vi "IRISS_FPGA_IO_v4.vi"() -> ()   [LabVIEW 2016]
doc: "This VI contains a basic quadrature decoder which is reset asynchronously upon clicking the reset button."
uses:
  <vilib>/Platform/TimedLoop/XDataNode/timing_clust.ctl
  <vilib>/Platform/TimedLoop/XDataNode/nitl_modes.ctl
  <vilib>/Platform/TimedLoop/XDataNode/wakeup.ctl
  <vilib>/rvi/Emulation/niFpgaGetClockAttributes.vi
  <vilib>/rvi/Emulation/niFpgaSctlEmulationGetInTimedLoop.vi
  <vilib>/rvi/Emulation/niFpgaEmulationReportErrorSimple.vi
  <vilib>/rvi/eio/common/nirviEmuTemplateMethod_errors.vi
  <vilib>/rvi/Emulation/niFpgaCriticalErrorInLSC.vi
  <vilib>/eio/EIONode/EIONode.xnode
  <vilib>/platform/TimedLoop/XDataNode/XDataNode.xnode
  <vilib>/Platform/TimedLoop/XDataNode/XDNodeRunTimeDep.lvlib
  Library/KevinLibraryAll/labview/KevLib01.lvlib
  Library/jmslib.lvlib
panel:
  in  "Connector2/DIO7":bool
  in  "Connector2/DIO8":bool
  in  "Connector2/DIO9":bool
  in  "Connector2/DIO10":bool
  in  "PWM1":fxp<+,32,0>
  in  "Period 1 (Ticks)":u32=1000
  in  "Period (Ticks)":u32=2000
  in  "DIR OCT Mot":bool
  in  "INHB OCT Mot":bool
  out "FAULT OCT Mot":bool
  out "Position OCT Mot":i32
  out "JumpBy2Error OCT Mot":i16
  in  "Reset OCT Mot":bool
  in  "OCT Mot DC":fxp<+,32,0>
  in  "Conn0/DIO15 Button 4":bool
  in  "Conn0/DIO12 Button 1":bool
  in  "Conn0/DIO13 Button 2":bool
  out "Home OCT z":bool
  in  "DIR Y":bool
  in  "INHB Y":bool
  out "FAULT Y":bool
  out "Position Y":i32
  out "JumpBy2Error Y":i16
  in  "Reset Y":bool
  in  "Y DC":fxp<+,32,0>
  in  "DIR X":bool
  in  "INHB X":bool
  out "FAULT X":bool
  out "Position X":i32
  out "JumpBy2Error X":i16
  in  "Reset X":bool
  in  "DIR Z":bool
  in  "INHB Z":bool
  out "FAULT Z":bool
  out "Position Z":i32
  out "JumpBy2Error Z":i16
  in  "Reset Z":bool
  in  "Z DC":fxp<+,32,0>
  in  "X DC":fxp<+,32,0>
  out "samples":i32
  out "Current Monitor":u32[](array[numeric])
  out "Raw Data Response (MSB)":bool[](array[boolean])
  out "Home L4":bool
  out "Home L1":bool
  out "Home L2":bool
  out "Home L3":bool
  in  "Positive Direction C1-4":bool
  out "JumpBy2Error C1-4":i16
  out "32 bit Position C1-4":i32
  in  "Reset C1-4":bool
  in  "Positive Direction C1-1":bool
  out "JumpBy2Error C1-1":i16
  out "32 bit Position C1-1":i32
  in  "Reset C1-1":bool
  out "32 bit Position 17":i32
  in  "Reset 17":bool
  in  "Positive Direction 17":bool
  out "JumpBy2Error 17":i16
  out "32 bit Position 16":i32
  in  "Reset 16":bool
  in  "Positive Direction 16":bool
  out "JumpBy2Error 16":i16
  out "32 bit Position 15":i32
  in  "Reset 15":bool
  in  "Positive Direction 15":bool
  out "JumpBy2Error 15":i16
  out "32 bit Position 14":i32
  in  "Reset 14":bool
  in  "Positive Direction 14":bool
  out "JumpBy2Error 14":i16
  out "32 bit Position 13":i32
  in  "Reset 13":bool
  in  "Positive Direction 13":bool
  out "JumpBy2Error 13":i16
  out "32 bit Position 12":i32
  in  "Reset 12":bool
  in  "Positive Direction 12":bool
  out "JumpBy2Error 12":i16
  out "32 bit Position 11":i32
  in  "Reset 11":bool
  in  "Positive Direction 11":bool
  out "JumpBy2Error 11":i16
  out "32 bit Position 10":i32
  in  "Reset 10":bool
  in  "Positive Direction 10":bool
  out "JumpBy2Error 10":i16
  out "32 bit Position 9":i32
  in  "Reset 9":bool
  in  "Positive Direction 9":bool
  out "JumpBy2Error 9":i16
  out "JumpBy2Error 3":i16
  in  "Positive Direction 3":bool
  out "JumpBy2Error 1":i16
  in  "Positive Direction 1":bool
  out "AI":i16[](array[numeric])
  out "32 bit Position 3":i32
  in  "Reset 3":bool
  in  "AO":i16[](array[numeric])=[0, 0, 0, 0, 0, 0, 0, 0]
  out "32 bit Position 1":i32
  in  "Reset 1":bool
  # "Accurus Buttons"
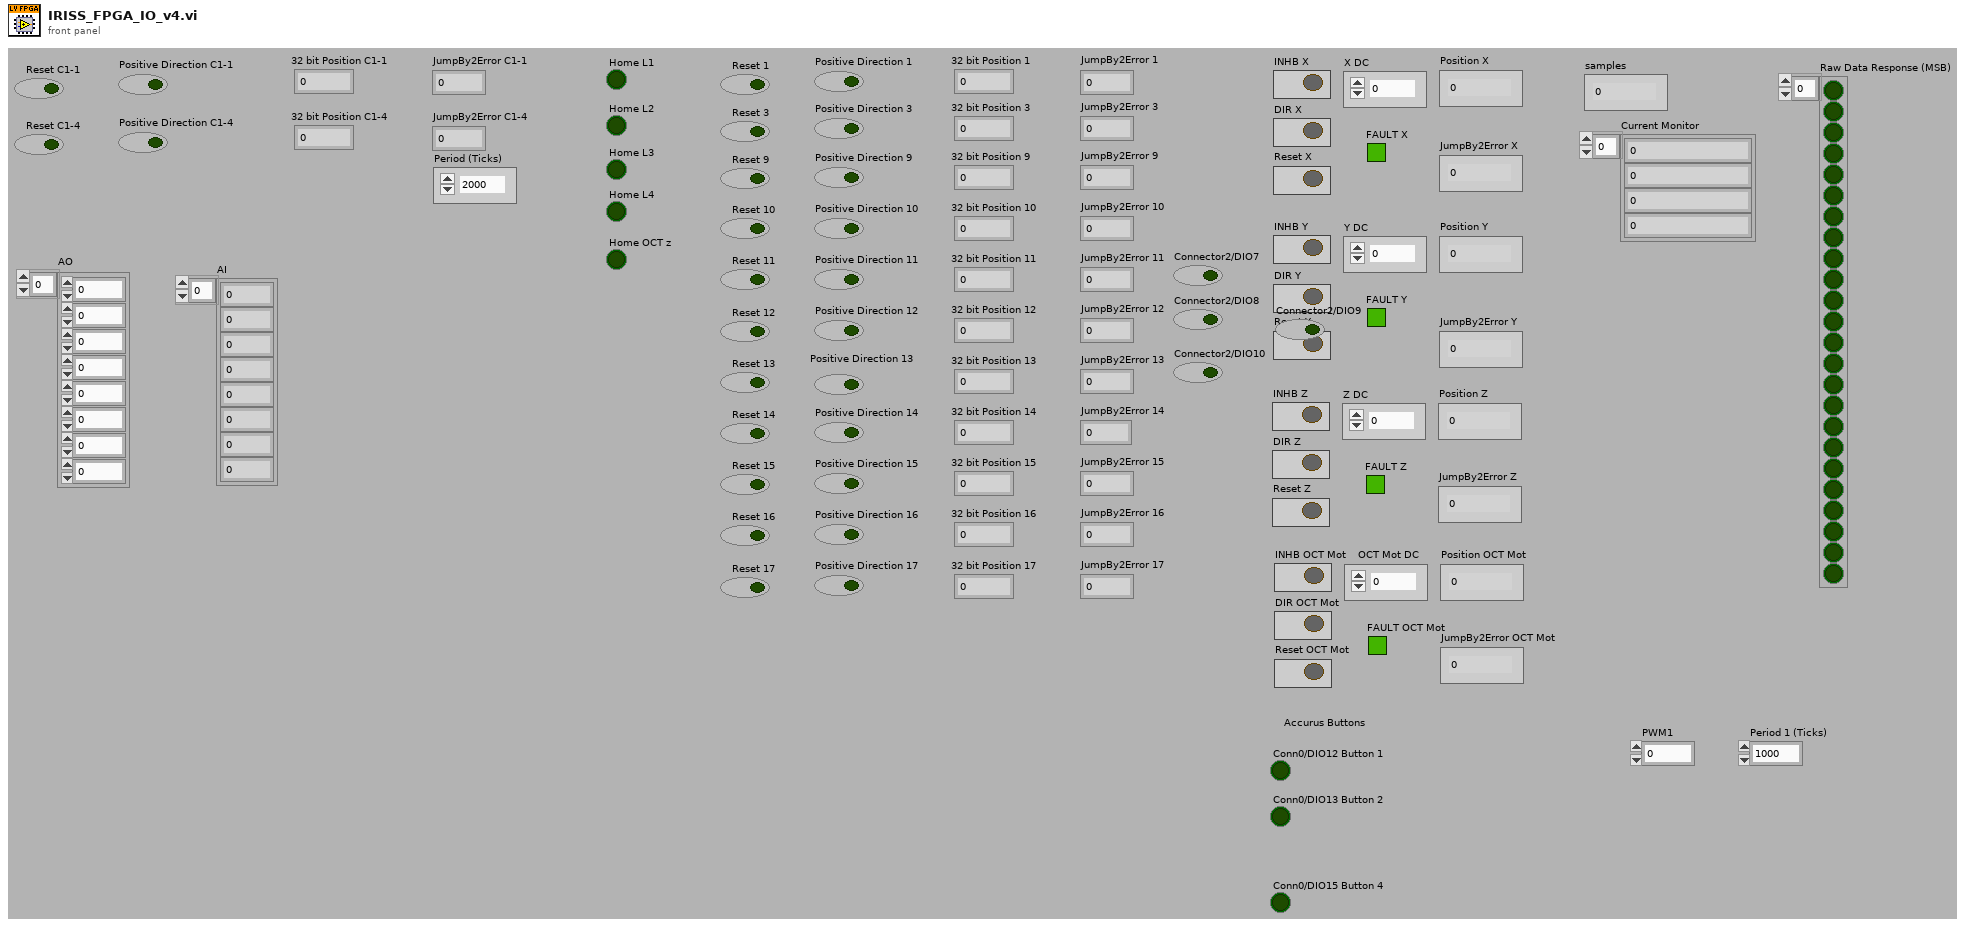
[diagram p1: front panel]
types:
  T1 = typedef "XDNodeRunTimeDep.lvlib/timing_clust.ctl" = cluster{"Expected End [f-1]":u64, "Actual End [f-1]":u64, "Finished Late? [f-1]":bool, "Expected End [i-1]":u64, "Actual End [i-1]":u64, "Finished Late? [i-1]":bool, "Expected Start [i]":u64, "Actual Start [i]":u64, "Expected Start [f]":u64, "Actual Start [f]":u64, "Source Name":string, "Structure Name":string, "Period":i64, "Deadline":i64, "Offset":i64, "Start":i64, "Priority":i32, "Timeout":i32, "Mode":T2, "Wakeup Reason":T3, "Error":errorcluster, "Source Type":string, "Secondary Source Type":string, "Global End Time":u64, "Global Start Time":u64, "Frame Duration":u64, "Iteration Duration":u64, "Assigned CPU":i32, "I/O Scan Engine Mode":u32}
  T2 = typedef "XDNodeRunTimeDep.lvlib/nitl_modes.ctl" = enum32{"No Change", "Process missed periods, maintain original phase", "Discard missed periods, maintain original phase", "Process missed periods, ignore original phase", "Discard missed periods, ignore original phase"}
  T3 = typedef "XDNodeRunTimeDep.lvlib/wakeup.ctl" = enum32{"Normal", "Aborted", "Asynchronous wakeup", "Timing source error", "Timed loop error", "Timeout"}
  T4 = cluster{"PWM In":refnum<k21>, "Direction":refnum<k21>, "Inhibit":refnum<k21>, "Encoder C":refnum<k21>, "Encoder B":refnum<k21>, "Encoder A":refnum<k21>, "Fault":refnum<k21>}
  T5 = cluster{"SCLK":refnum<k21>, "MOSI":refnum<k21>, "MISO":refnum<k21>}
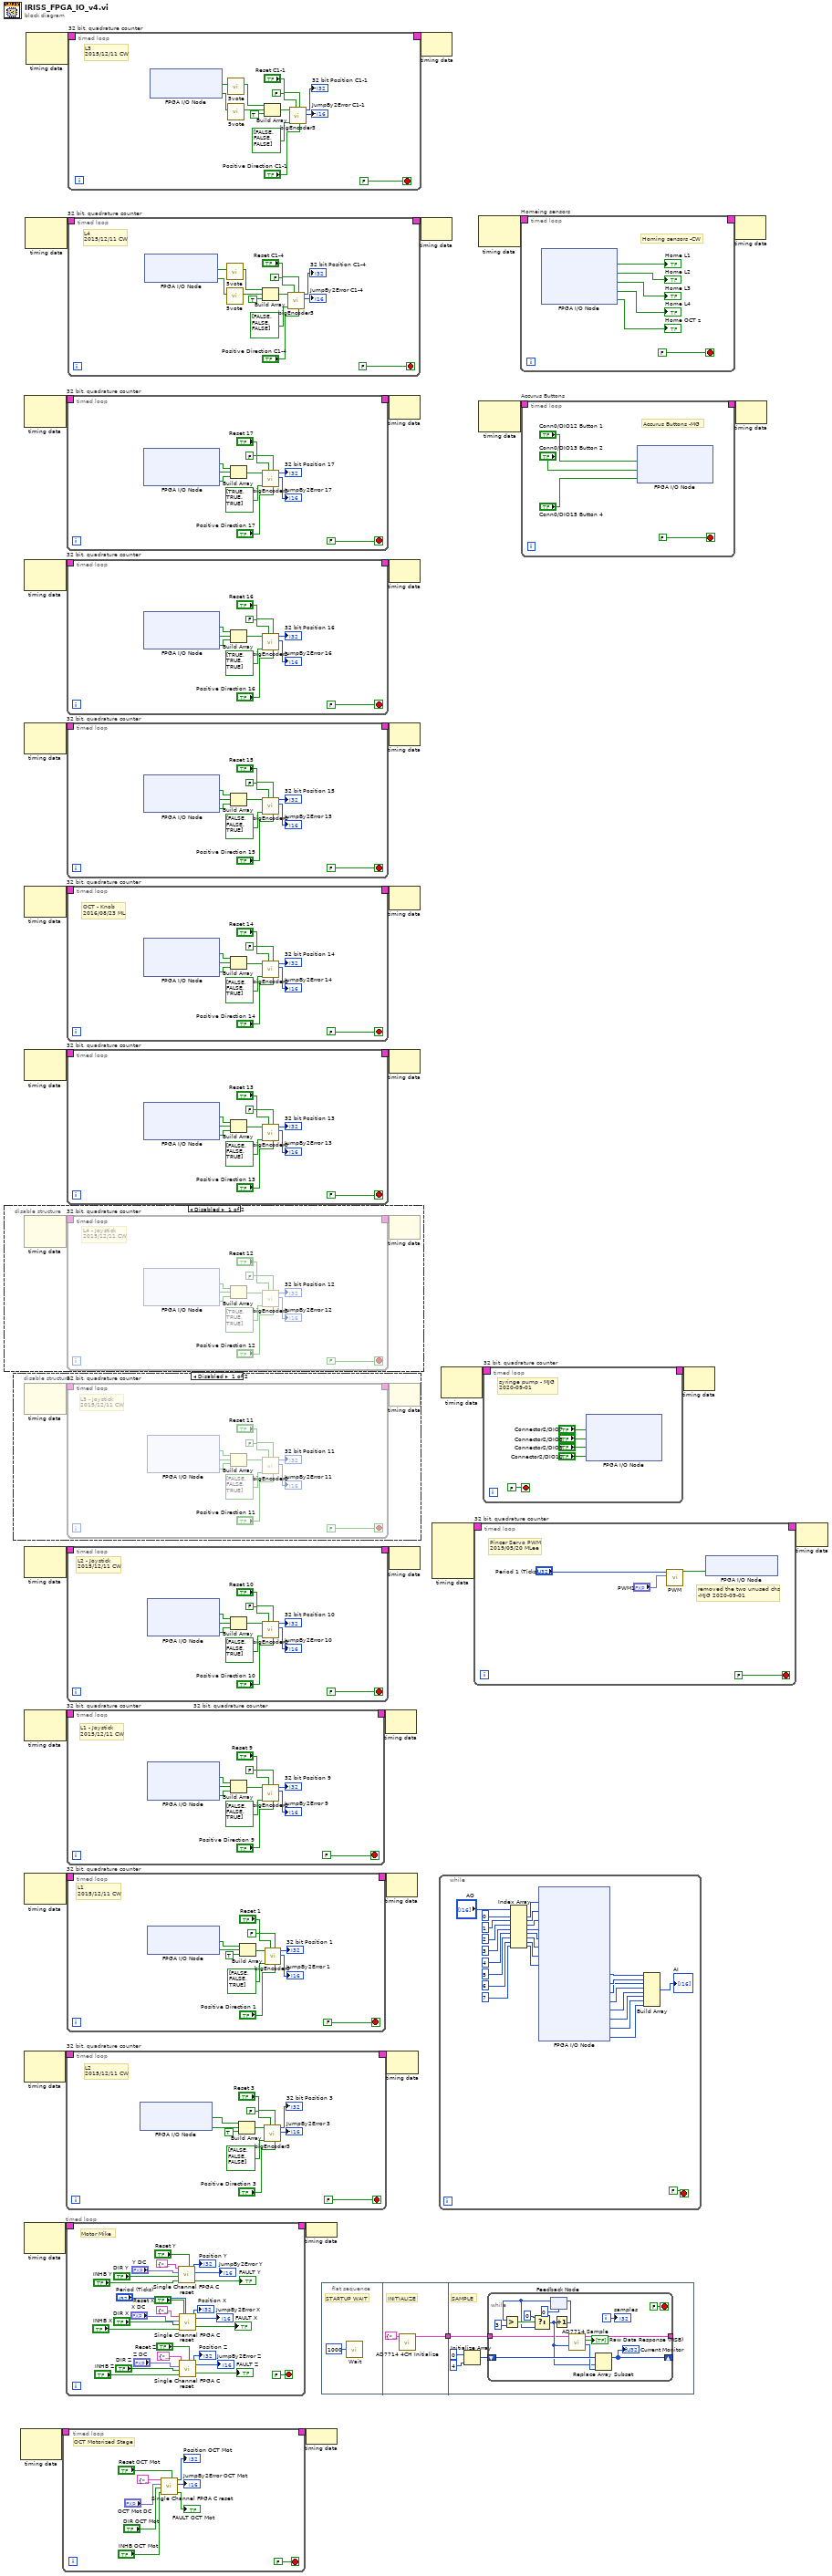
[diagram p0: block diagram]
diagram:
  n1 = disable-structure shown="Disabled" {
    frame Disabled {
      n2 = node-c288() -> (w37:T1)  [unwired: 2 out]
      n3 = timed-loop "32 bit, quadrature counter" {
        timing-out: [_] -> w36
        timing: w37 -> [_]
        stop <- FALSE stop-if-true
        # "L4 - Joystick\n2015/12/11 CW"
        n4 = xnode "FPGA I/O Node"() -> ("Connector2/DIO9"=w47:bool, "Connector2/DIO10"=w46:bool, "Connector2/DIO11"=w38:bool)  [unwired: 3 in, 3 out]
        n5 = Build Array(w47, w46, w38) -> (w45:bool[])
        n6 = call "bigEncoder3.vi"("Positive Direction"="Positive Direction 12", "ForceReset"="Reset 12", "Allow C Reset?"=FALSE, "Reset Array"=bool[] [TRUE, TRUE, TRUE], "Encoder Array"=w45) -> ("JumpBy2Error"=→"JumpBy2Error 12":i16, "Position"=→"32 bit Position 12":i32)  [unwired: 5 out]
      }
      n7 = node-c288(w36) -> ()  [unwired: 1 out]
    }
    frame Enabled {
    }
  }
  n8 = disable-structure shown="Disabled" {
    frame Disabled {
      n9 = node-c288() -> (w54:T1)  [unwired: 2 out]
      n10 = timed-loop "32 bit, quadrature counter" {
        timing-out: [_] -> w53
        timing: w54 -> [_]
        stop <- FALSE stop-if-true
        # "L3 - Joystick\n2015/12/11 CW"
        n11 = xnode "FPGA I/O Node"() -> ("Connector2/DIO6"=w64:bool, "Connector2/DIO7"=w63:bool, "Connector2/DIO8"=w55:bool)  [unwired: 3 in, 3 out]
        n12 = Build Array(w64, w63, w55) -> (w62:bool[])
        n13 = call "bigEncoder3.vi"("Positive Direction"="Positive Direction 11", "ForceReset"="Reset 11", "Allow C Reset?"=FALSE, "Reset Array"=bool[] [FALSE, FALSE, TRUE], "Encoder Array"=w62) -> ("JumpBy2Error"=→"JumpBy2Error 11":i16, "Position"=→"32 bit Position 11":i32)  [unwired: 5 out]
      }
      n14 = node-c288(w53) -> ()  [unwired: 1 out]
    }
    frame Enabled {
    }
  }
  n15 = node-c288() -> (w8:T1)  [unwired: 2 in]
  n16 = node-c288() -> (w33:T1)  [unwired: 2 out]
  n17 = node-c288() -> (w13:T1)  [unwired: 2 in]
  n18 = node-c288() -> (w21:T1)  [unwired: 2 out]
  n19 = node-c288() -> (w23:T1)  [unwired: 2 out]
  n20 = node-c288() -> (w25:T1)  [unwired: 2 out]
  n21 = node-c288() -> (w27:T1)  [unwired: 2 out]
  n22 = node-c288() -> (w29:T1)  [unwired: 2 out]
  n23 = node-c288() -> (w2:T1)  [unwired: 2 out]
  n24 = node-c288() -> (w31:T1)  [unwired: 2 out]
  n25 = node-c288() -> (w34:T1)  [unwired: 2 out]
  n26 = node-c288() -> (w17:T1)  [unwired: 2 out]
  n27 = node-c288() -> (w19:T1)  [unwired: 2 out]
  n28 = timed-loop {
    timing: w8 -> [_]
    timing-out: [_] -> w7
    stop <- FALSE stop-if-true
    # "OCT Motorized Stage"
    n29 = call "Single Channel FPGA C reset.vi"("Reset"="Reset OCT Mot", "INHB"="INHB OCT Mot", "DIR"="DIR OCT Mot", "Duty"="OCT Mot DC", "IO Channels"=T4 {"PWM In"="Connector1/DIO7", "Direction"="Connector1/DIO8", "Inhibit"="Connector1/DIO9", "Encoder C"="Connector1/DIO10", "Encoder B"="Connector1/DIO11", "Encoder A"="Connector1/DIO12", "Fault"="Connector1/DIO13"}) -> ("FAULT"=→"FAULT OCT Mot":bool, "JumpBy2Error"=→"JumpBy2Error OCT Mot":i16, "Position"=→"Position OCT Mot":i32)  [unwired: 4 in]
  }
  n30 = timed-loop "32 bit, quadrature counter" {
    timing-out: [_] -> w32
    timing: w33 -> [_]
    stop <- FALSE stop-if-true
    # "L2\n2015/12/11 CW"
    n31 = xnode "FPGA I/O Node"() -> ("Connector0/DIO2"=w84:bool, "Connector0/DIO3"=w83:bool)  [unwired: 2 in, 2 out]
    n32 = Build Array(w84, w83, TRUE ("element")) -> (w90:bool[])
    n33 = call "bigEncoder3.vi"("Positive Direction"="Positive Direction 3", "ForceReset"="Reset 3", "Allow C Reset?"=FALSE, "Reset Array"=bool[] [FALSE, FALSE, FALSE], "Encoder Array"=w90) -> ("JumpBy2Error"=→"JumpBy2Error 3":i16, "Position"=→"32 bit Position 3":i32)  [unwired: 5 out]
  }
  n34 = timed-loop {
    timing: w13 -> [_]
    timing-out: [_] -> w12
    stop <- FALSE stop-if-true
    # "Motor Mike"
    n35 = call "Single Channel FPGA C reset.vi"("Reset"="Reset Y", "INHB"="INHB Y", "DIR"="DIR Y", "Duty"="Y DC", "IO Channels"=T4 {"PWM In"="Connector1/DIO1", "Direction"="Connector1/DIO2", "Inhibit"="Connector1/DIO3", "Encoder C"="Connector1/DIO4", "Encoder B"="Connector1/DIO5", "Encoder A"="Connector1/DIO6", "Fault"="Connector1/DIO0"}) -> ("FAULT"=→"FAULT Y":bool, "JumpBy2Error"=→"JumpBy2Error Y":i16, "Position"=→"Position Y":i32)  [unwired: 4 in]
    n36 = call "Single Channel FPGA C reset.vi"("Reset"="Reset X", "Period (Ticks)"="Period (Ticks)", "INHB"="INHB X", "DIR"="DIR X", "Duty"="X DC", "IO Channels"=T4 {"PWM In"="Connector1/DIO20", "Direction"="Connector1/DIO21", "Inhibit"="Connector1/DIO22", "Encoder C"="Connector1/DIO23", "Encoder B"="Connector1/DIO24", "Encoder A"="Connector1/DIO25", "Fault"="Connector1/DIO27"}) -> ("FAULT"=→"FAULT X":bool, "JumpBy2Error"=→"JumpBy2Error X":i16, "Position"=→"Position X":i32)  [unwired: 3 in]
    n37 = call "Single Channel FPGA C reset.vi"("Reset"="Reset Z", "INHB"="INHB Z", "DIR"="DIR Z", "Duty"="Z DC", "IO Channels"=T4 {"PWM In"="Connector1/DIO14", "Direction"="Connector1/DIO15", "Inhibit"="Connector1/DIO16", "Encoder C"="Connector1/DIO17", "Encoder B"="Connector1/DIO18", "Encoder A"="Connector1/DIO19", "Fault"="Connector1/DIO26"}) -> ("FAULT"=→"FAULT Z":bool, "JumpBy2Error"=→"JumpBy2Error Z":i16, "Position"=→"Position Z":i32)  [unwired: 4 in]
  }
  n38 = timed-loop "32 bit, quadrature counter" {
    timing-out: [_] -> w20
    timing: w21 -> [_]
    stop <- FALSE stop-if-true
    n39 = xnode "FPGA I/O Node"() -> ("Connector2/DIO24"=w131:bool, "Connector2/DIO25"=w130:bool, "Connector2/DIO26"=w122:bool)  [unwired: 3 in, 3 out]
    n40 = Build Array(w131, w130, w122) -> (w129:bool[])
    n41 = call "bigEncoder3.vi"("Positive Direction"="Positive Direction 17", "ForceReset"="Reset 17", "Allow C Reset?"=FALSE, "Reset Array"=bool[] [TRUE, TRUE, TRUE], "Encoder Array"=w129) -> ("JumpBy2Error"=→"JumpBy2Error 17":i16, "Position"=→"32 bit Position 17":i32)  [unwired: 5 out]
  }
  n42 = timed-loop "32 bit, quadrature counter" {
    timing-out: [_] -> w22
    timing: w23 -> [_]
    stop <- FALSE stop-if-true
    n43 = xnode "FPGA I/O Node"() -> ("Connector2/DIO21"=w144:bool, "Connector2/DIO22"=w143:bool, "Connector2/DIO23"=w135:bool)  [unwired: 3 in, 3 out]
    n44 = Build Array(w144, w143, w135) -> (w142:bool[])
    n45 = call "bigEncoder3.vi"("Positive Direction"="Positive Direction 16", "ForceReset"="Reset 16", "Allow C Reset?"=FALSE, "Reset Array"=bool[] [TRUE, TRUE, TRUE], "Encoder Array"=w142) -> ("JumpBy2Error"=→"JumpBy2Error 16":i16, "Position"=→"32 bit Position 16":i32)  [unwired: 5 out]
  }
  n46 = timed-loop "32 bit, quadrature counter" {
    timing-out: [_] -> w24
    timing: w25 -> [_]
    stop <- FALSE stop-if-true
    n47 = xnode "FPGA I/O Node"() -> ("Connector2/DIO18"=w157:bool, "Connector2/DIO19"=w156:bool, "Connector2/DIO20"=w148:bool)  [unwired: 3 in, 3 out]
    n48 = Build Array(w157, w156, w148) -> (w155:bool[])
    n49 = call "bigEncoder3.vi"("Positive Direction"="Positive Direction 15", "ForceReset"="Reset 15", "Allow C Reset?"=FALSE, "Reset Array"=bool[] [FALSE, FALSE, TRUE], "Encoder Array"=w155) -> ("JumpBy2Error"=→"JumpBy2Error 15":i16, "Position"=→"32 bit Position 15":i32)  [unwired: 5 out]
  }
  n50 = timed-loop "32 bit, quadrature counter" {
    timing-out: [_] -> w26
    timing: w27 -> [_]
    stop <- FALSE stop-if-true
    # "OCT - Knob\n2016/08/23 ML"
    n51 = xnode "FPGA I/O Node"() -> ("Connector2/DIO15"=w170:bool, "Connector2/DIO16"=w169:bool, "Connector2/DIO17"=w161:bool)  [unwired: 3 in, 3 out]
    n52 = Build Array(w170, w169, w161) -> (w168:bool[])
    n53 = call "bigEncoder3.vi"("Positive Direction"="Positive Direction 14", "ForceReset"="Reset 14", "Allow C Reset?"=FALSE, "Reset Array"=bool[] [FALSE, FALSE, TRUE], "Encoder Array"=w168) -> ("JumpBy2Error"=→"JumpBy2Error 14":i16, "Position"=→"32 bit Position 14":i32)  [unwired: 5 out]
  }
  n54 = timed-loop "32 bit, quadrature counter" {
    timing-out: [_] -> w28
    timing: w29 -> [_]
    stop <- FALSE stop-if-true
    n55 = xnode "FPGA I/O Node"() -> ("Connector2/DIO12"=w183:bool, "Connector2/DIO13"=w182:bool, "Connector2/DIO14"=w174:bool)  [unwired: 3 in, 3 out]
    n56 = Build Array(w183, w182, w174) -> (w181:bool[])
    n57 = call "bigEncoder3.vi"("Positive Direction"="Positive Direction 13", "ForceReset"="Reset 13", "Allow C Reset?"=FALSE, "Reset Array"=bool[] [FALSE, FALSE, TRUE], "Encoder Array"=w181) -> ("JumpBy2Error"=→"JumpBy2Error 13":i16, "Position"=→"32 bit Position 13":i32)  [unwired: 5 out]
  }
  n58 = timed-loop "32 bit, quadrature counter" {
    timing-out: [_] -> w1
    timing: w2 -> [_]
    stop <- FALSE stop-if-true
    # "L2 - Joystick\n2015/12/11 CW"
    n59 = xnode "FPGA I/O Node"() -> ("Connector2/DIO3"=w196:bool, "Connector2/DIO4"=w195:bool, "Connector2/DIO5"=w187:bool)  [unwired: 3 in, 3 out]
    n60 = Build Array(w196, w195, w187) -> (w194:bool[])
    n61 = call "bigEncoder3.vi"("Positive Direction"="Positive Direction 10", "ForceReset"="Reset 10", "Allow C Reset?"=FALSE, "Reset Array"=bool[] [FALSE, FALSE, TRUE], "Encoder Array"=w194) -> ("JumpBy2Error"=→"JumpBy2Error 10":i16, "Position"=→"32 bit Position 10":i32)  [unwired: 5 out]
  }
  n62 = timed-loop "32 bit, quadrature counter" {
    timing-out: [_] -> w30
    timing: w31 -> [_]
    stop <- FALSE stop-if-true
    # "L1 - Joystick\n2015/12/11 CW"
    n63 = xnode "FPGA I/O Node"() -> ("Connector2/DIO0"=w209:bool, "Connector2/DIO1"=w208:bool, "Connector2/DIO2"=w200:bool)  [unwired: 3 in, 3 out]
    n64 = Build Array(w209, w208, w200) -> (w207:bool[])
    n65 = call "bigEncoder3.vi"("Positive Direction"="Positive Direction 9", "ForceReset"="Reset 9", "Allow C Reset?"=FALSE, "Reset Array"=bool[] [FALSE, FALSE, TRUE], "Encoder Array"=w207) -> ("JumpBy2Error"=→"JumpBy2Error 9":i16, "Position"=→"32 bit Position 9":i32)  [unwired: 5 out]
  }
  n66 = timed-loop "32 bit, quadrature counter" {
    timing-out: [_] -> w35
    timing: w34 -> [_]
    stop <- FALSE stop-if-true
    # "L1\n2015/12/11 CW"
    n67 = xnode "FPGA I/O Node"() -> ("Connector0/DIO0"=w222:bool, "Connector0/DIO1"=w221:bool)  [unwired: 2 in, 2 out]
    n68 = Build Array(w222, w221, TRUE ("element")) -> (w220:bool[])
    n69 = call "bigEncoder3.vi"("Positive Direction"="Positive Direction 1", "ForceReset"="Reset 1", "Allow C Reset?"=FALSE, "Reset Array"=bool[] [FALSE, FALSE, TRUE], "Encoder Array"=w220) -> ("JumpBy2Error"=→"JumpBy2Error 1":i16, "Position"=→"32 bit Position 1":i32)  [unwired: 5 out]
  }
  n70 = timed-loop "32 bit, quadrature counter" {
    timing-out: [_] -> w16
    timing: w17 -> [_]
    stop <- FALSE stop-if-true
    # "L4\n2015/12/11 CW"
    n71 = xnode "FPGA I/O Node"() -> ("Connector0/DIO6"=w229:bool, "Connector0/DIO7"=w228:bool)  [unwired: 2 in, 2 out]
    n72 = call "5vote.vi"("Input"=w229) -> ("vote5"=w226:bool)  [unwired: 10 in]
    n73 = call "5vote.vi"("Input"=w228) -> ("vote5"=w227:bool)  [unwired: 10 in]
    n74 = Build Array(w226, w227, TRUE ("element")) -> (w237:bool[])
    n75 = call "bigEncoder3.vi"("Positive Direction"="Positive Direction C1-4", "ForceReset"="Reset C1-4", "Allow C Reset?"=FALSE, "Reset Array"=bool[] [FALSE, FALSE, FALSE], "Encoder Array"=w237) -> ("JumpBy2Error"=→"JumpBy2Error C1-4":i16, "Position"=→"32 bit Position C1-4":i32)  [unwired: 5 out]
  }
  n76 = timed-loop "32 bit, quadrature counter" {
    timing-out: [_] -> w18
    timing: w19 -> [_]
    stop <- FALSE stop-if-true
    # "L3\n2015/12/11 CW"
    n77 = xnode "FPGA I/O Node"() -> ("Connector0/DIO4"=w244:bool, "Connector0/DIO5"=w243:bool)  [unwired: 2 in, 2 out]
    n78 = call "5vote.vi"("Input"=w244) -> ("vote5"=w241:bool)  [unwired: 10 in]
    n79 = call "5vote.vi"("Input"=w243) -> ("vote5"=w242:bool)  [unwired: 10 in]
    n80 = Build Array(w241, w242, TRUE ("element")) -> (w252:bool[])
    n81 = call "bigEncoder3.vi"("Positive Direction"="Positive Direction C1-1", "ForceReset"="Reset C1-1", "Allow C Reset?"=FALSE, "Reset Array"=bool[] [FALSE, FALSE, FALSE], "Encoder Array"=w252) -> ("JumpBy2Error"=→"JumpBy2Error C1-1":i16, "Position"=→"32 bit Position C1-1":i32)  [unwired: 5 out]
  }
  n82 = node-c288(w12) -> ()
  n83 = node-c288(w7) -> ()
  n84 = flat-sequence {
    tunnel: [w257] -> w11
    tunnel: w11 -> [w259]
    frame #0 {
      # "STARTUP WAIT"
      n85 = call "Wait"("Count(uSec)"=u32 1000) -> ()  [unwired: 1 out]
    }
    frame #1 {
      # "INITIALIZE"
      n86 = call "AD7714 4CH Initialize.vi"("I/O Cluster In"=T5 {"SCLK"="Connector1/DIO29", "MOSI"="Connector1/DIO35", "MISO"="Connector1/DIO31"}) -> ("I/O Cluster Out"=w257:T5)  [unwired: 10 in]
    }
    frame #2 {
      # "SAMPLE"
      n87 = Initialize Array(u32 0, 4 ("dimension size")) -> (w260:u32[])
      n88 = while {
        shift-right: [w268] -> _
        shift-left: w260 -> [w269]
        tunnel: w259 -> [w265]
        tunnel: [w264] -> _
        i -> [w276]
        stop <- FALSE stop-if-true
        n89 = feedback #1(i16 0) -> (w272:i16)
        n90 = Greater?(x=w272, y=i16 3) -> (0:w273:bool)
        n91 = Select(t=i16 0, s=w273, f=w272) -> (s? t:f=w266:i16)
        n92 = Increment(x=w266) -> (x+1=w270:i16)
        n93 = feedback-in #1(w270) -> ()
        n94 = call "AD7714 Sample.vi"("Channel"=w266, "I/O Cluster In"=w265) -> ("Data"=w267:u32, "Raw Data Response (MSB)"=→"Raw Data Response (MSB)":bool[], "I/O Cluster Out"=w264:T5)  [unwired: 7 in]
        n95 = Replace Array Subset(array=w269, new element=w267, index=w266) -> (w268:u32[])
        "Current Monitor" <- w268
        "samples" <- w276
      }
    }
  }
  n96 = node-c288(w30) -> ()  [unwired: 1 out]
  n97 = node-c288(w35) -> ()  [unwired: 1 out]
  n98 = node-c288(w32) -> ()  [unwired: 1 out]
  n99 = node-c288(w20) -> ()  [unwired: 1 out]
  n100 = node-c288(w22) -> ()  [unwired: 1 out]
  n101 = node-c288(w24) -> ()  [unwired: 1 out]
  n102 = node-c288(w26) -> ()  [unwired: 1 out]
  n103 = node-c288(w28) -> ()  [unwired: 1 out]
  n104 = node-c288(w1) -> ()  [unwired: 1 out]
  n105 = node-c288(w16) -> ()  [unwired: 1 out]
  n106 = node-c288(w18) -> ()  [unwired: 1 out]
  n107 = node-c288() -> (w6:T1)  [unwired: 4 in, 1 out]
  n108 = while {
    stop <- FALSE stop-if-true
    n109 = Index Array(array="AO", index #1=0 ("index"), index #2=1 ("index"), index #3=2 ("index"), index #4=3 ("index"), index #5=4 ("index"), index #6=5 ("index"), index #7=6 ("index"), index #8=7 ("index")) -> (element #1=w295:i16, element #2=w294:i16, element #3=w293:i16, element #4=w292:i16, element #5=w291:i16, element #6=w290:i16, element #7=w289:i16, element #8=w288:i16)
    n110 = xnode "FPGA I/O Node"("Connector0/AO0"=w295, "Connector0/AO1"=w294, "Connector0/AO2"=w293, "Connector0/AO3"=w292, "Connector0/AO4"=w291, "Connector0/AO5"=w290, "Connector0/AO6"=w289, "Connector0/AO7"=w288) -> ("Connector0/AI0"=w286:i16, "Connector0/AI1"=w285:i16, "Connector0/AI2"=w283:i16, "Connector0/AI3"=w282:i16, "Connector0/AI4"=w281:i16, "Connector0/AI5"=w280:i16, "Connector0/AI6"=w279:i16, "Connector0/AI7"=w278:i16)  [unwired: 16 in, 16 out]
    n111 = Build Array(w286, w285, w283, w282, w281, w280, w279, w278) -> (→"AI":i16[])
  }
  n112 = node-c288() -> (w4:T1)  [unwired: 2 out]
  n113 = timed-loop "32 bit, quadrature counter" {
    timing-out: [_] -> w5
    timing: w6 -> [_]
    stop <- FALSE stop-if-true
    # "removed the two unused chs\n-MJG 2020-09-01"
    # "Pincer Servo PWM\n2019/05/20 MLee"
    n114 = call "PWM.vi"("Duty Cycle"="PWM1", "Period (Ticks)"="Period 1 (Ticks)") -> ("PWM Out"=w307:bool)  [unwired: 8 in, 1 out]
    n115 = xnode "FPGA I/O Node"("Connector2/DIO6"=w307) -> ()  [unwired: 1 in, 1 out]
  }
  n116 = node-c288() -> (w15:T1)  [unwired: 2 out]
  n117 = node-c288() -> (w10:T1)  [unwired: 2 out]
  n118 = timed-loop "32 bit, quadrature counter" {
    timing-out: [_] -> w3
    timing: w4 -> [_]
    stop <- FALSE stop-if-true
    # "syringe pump - MJG \n2020-09-01"
    n119 = xnode "FPGA I/O Node"("Connector2/DIO7"="Connector2/DIO7", "Connector2/DIO8"="Connector2/DIO8", "Connector2/DIO9"="Connector2/DIO9", "Connector2/DIO10"="Connector2/DIO10") -> ()  [unwired: 4 in, 4 out]
  }
  n120 = timed-loop "Homeing sensors" {
    timing-out: [_] -> w14
    timing: w15 -> [_]
    stop <- FALSE stop-if-true
    # "Homing sensors -CW"
    n121 = xnode "FPGA I/O Node"() -> ("Connector0/DIO8"=→"Home L1":bool, "Connector0/DIO9"=→"Home L2":bool, "Connector0/DIO10"=→"Home L3":bool, "Connector0/DIO11"=→"Home L4":bool, "Connector0/DIO14"=→"Home OCT z":bool)  [unwired: 5 in, 5 out]
  }
  n122 = timed-loop "Accurus Buttons" {
    timing-out: [_] -> w9
    timing: w10 -> [_]
    stop <- FALSE stop-if-true
    # "Accurus Buttons -MG"
    n123 = xnode "FPGA I/O Node"("Connector0/DIO12"="Conn0/DIO12 Button 1", "Connector0/DIO13"="Conn0/DIO13 Button 2", "Connector0/DIO15"="Conn0/DIO15 Button 4") -> ()  [unwired: 3 in, 3 out]
  }
  n124 = node-c288(w3) -> ()  [unwired: 1 out]
  n125 = node-c288(w14) -> ()  [unwired: 1 out]
  n126 = node-c288(w9) -> ()  [unwired: 1 out]
  n127 = node-c288(w5) -> ()  [unwired: 1 out]
